vi "Test Get Code Coverage Ignores Framework.vi"(8 "error in (no error)":errorcluster, 11 "Test Case In":refnum<class "Coverage Test.lvclass">) -> (0 "error out":errorcluster, 3 "Test Case Out":refnum<class "Coverage Test.lvclass">)   [LabVIEW 2020, in "LUnit Tests.lvlib" / "Coverage Test.lvclass"]
uses:
  Coverage Test.lvclass
  Coverage Test.lvclass/Coverage Test.ctl
  01074fa8-ee8a-411d-bc8b-fc92c4f90959.vi
  source/Framework/Coverage Analyzer/Coverage Analyzer.lvclass
  Test Dummys/Test Case Test Double/Test Case Test Double.lvclass
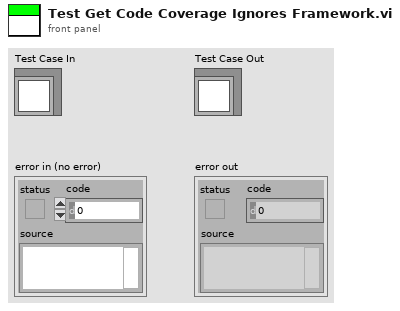
[diagram p1: front panel]
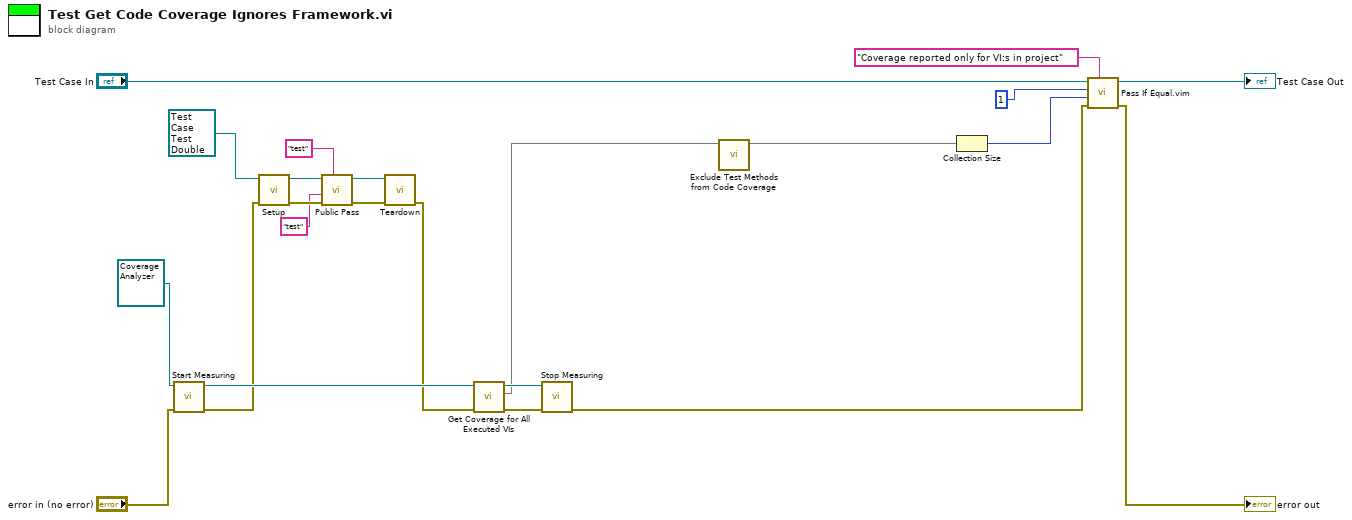
[diagram p0: block diagram]
diagram:
  n1 = call "Start Measuring.vi"("error in (no error)"="error in (no error)", "Coverage Analyzer in"=refnum<class "Coverage Analyzer.lvclass"> refnum) -> ("error out"=w3:errorcluster, "Coverage Analyzer out"=w15:refnum<class "Coverage Analyzer.lvclass">)  [unwired: 8 in]
  n2 = call-dynamic "Setup.vi"("error in (no error)"=w3, "LUnit Test Case In"=refnum<class "Test Case Test Double.lvclass"> refnum ("Test Case Test Double in")) -> ("error out"=w9:errorcluster, "LUnit Test Case Out"=w5:refnum<class "Test Case Test Double.lvclass">)  [unwired: 8 in]
  n3 = call "Public Pass.vi"("Description"="test", "error in (no error)"=w9, "Message"="test", "Test Case Test Double in"=w5) -> ("error out"=w7:errorcluster, "Test Case Test Double out"=w8:refnum<class "Test Case Test Double.lvclass">)  [unwired: 6 in]
  n4 = call-dynamic "Teardown.vi"("error in (no error)"=w7, "LUnit Test Case In"=w8) -> ("error out"=w4:errorcluster)  [unwired: 8 in, 1 out]
  n5 = call "Get Coverage for All Executed VIs.vi"("error in (no error)"=w4, "Coverage Analyzer in"=w15) -> ("error out"=w16:errorcluster, "Code Coverage"=w12:map{path, dbl}, "Coverage Analyzer out"=w14:refnum<class "Coverage Analyzer.lvclass">)  [unwired: 7 in]
  n6 = call "Stop Measuring.vi"("error in (no error)"=w16, "Coverage Analyzer in"=w14) -> ("error out"=w18:errorcluster)  [unwired: 8 in, 1 out]
  n7 = call "Exclude Test Methods from Code Coverage.vi"("Code Coverage"=w12) -> ("Filtered Code Coverage"=w11:map{path, dbl})  [unwired: 10 in]
  n8 = Collection Size(1:w11) -> (0:w10:i32)
  n9 = call "Pass If Equal.vim"("Description"="Coverage reported only for VI:s in project", "error in (no error)"=w18, "Actual"=w10, "Expected"=1 ("size"), "LUnit Test Case In"="Test Case In") -> ("error out"=→"error out":errorcluster, "LUnit Test Case Out"=→"Test Case Out":refnum<class "Coverage Test.lvclass">)  [unwired: 5 in]
